vi "GenerateWaveformforwavefirngraph.vi"() -> (1 "Waveform Graph":dbl[][](graph))   [LabVIEW 2012]
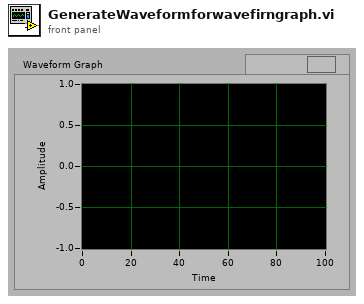
[diagram p1: front panel]
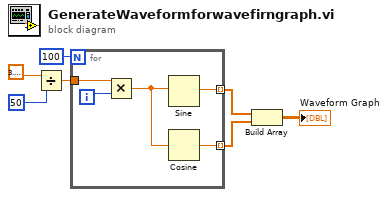
[diagram p0: block diagram]
diagram:
  n1 = Divide(x=3.141592653589793, y=50) -> (x/y=w5:dbl)
  n2 = for {
    N: 100 -> [_]
    tunnel: w5 -> [w12]
    tunnel: [w9] -> w2 mode=indexing
    tunnel: [w8] -> w1 mode=indexing
    i -> [w11]
    n3 = Multiply(x=w12, y=w11) -> (x*y=w10:dbl)
    n4 = Sine(x=w10) -> (sin(x)=w9:dbl)
    n5 = Cosine(x=w10) -> (cos(x)=w8:dbl)
  }
  n6 = Build Array(w2, w1) -> (→"Waveform Graph":dbl[][])
